vi "MainProgram.vi"() -> ()   [LabVIEW 2012]
uses:
  <vilib>/vision/Image Controls.llb/IMAQ Image.ctl
panel:
  out "error out 3":errorcluster
  out "error out 2":errorcluster
  out "error out":errorcluster
  in  "Tab Control":enum32{"MainProgram", ""}(tab)
  in  "Start Button":bool
  out "Judgment Failed":bool
  out "Image Out 2":T1(plugin-control)
  out "Red Found":i32
  out "R Score":sgl
  out "Red Status":bool
  in  "R Min Score":sgl=650.0
  in  "R Upper":dbl
  in  "R Lower":dbl
  in  "G Min score":sgl=800.0
  in  "G Upper":dbl
  in  "G Lower":dbl
  out "Green Status":bool
  out "G Score":sgl
  out "Green Found":i32
  out "Blue Status":bool
  out "Blue Found":i32
  out "B Score":sgl
  in  "B Min score":sgl=650.0
  in  "B Upper":dbl
  in  "B Lower":dbl
  out "Yellow Status":bool
  out "Yellow Found":i32
  out "Y Score":sgl
  in  "Y Min score":sgl=650.0
  in  "Y Upper":dbl
  in  "Y Lower":dbl
  out "Judgment Passed":bool
  in  "Stop (F)":bool
  out "Image Out 4":T1
  out "Image Out":T1(plugin-control)
  # "Check Fuse (Ver.1)"
  # "Test Result"
  # "Pass"
  # "Fail"
  # "Red Fuse"
  # "Green Fuse"
  # "Blue Fuse"
  # "Yellow Fuse"
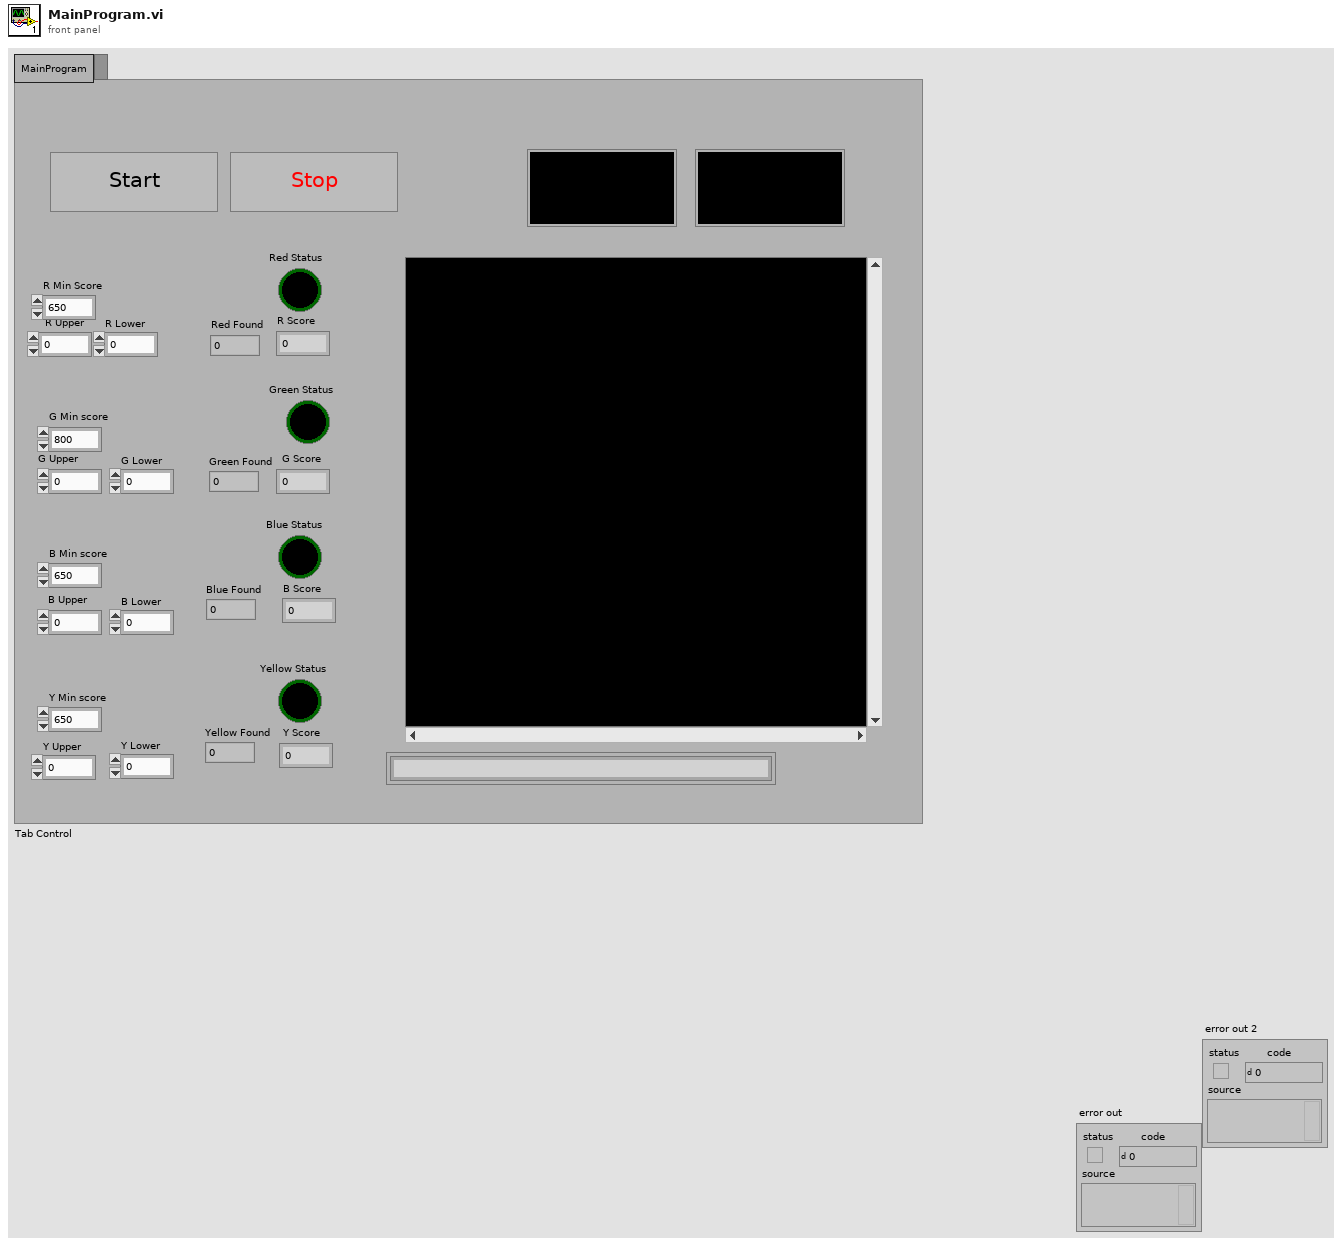
[diagram p1: front panel]
types:
  T1 = typedef "IMAQ Image.ctl" = refnum<image>
  T2 = cluster{"Desired Font (Application)":enum16{"User-specified Font", "Application Font", "System Font", "Dialog Font"}, "[User-specified Font]":cluster{"Font Name":string, "Size":i16, "Strikeout?":bool, "Italic?":bool, "Underline?":bool, "Outline?":bool, "Shadow?":bool, "Bold?":bool, "Rotation Angle":dbl}, "Horizontal Alignment":i16, "Vertical Alignment":i16}
  T3 = cluster{"Position":cluster{"x":sgl, "y":sgl}, "Angle":sgl, "Scale":sgl, "Score":sgl, "Bounding Box":cluster{"x":sgl, "y":sgl}[]}[]
  T4 = cluster{"Position":cluster{"x":sgl, "y":sgl}, "Angle":sgl, "Scale":sgl, "Score":sgl, "Bounding Box":cluster{"x":sgl, "y":sgl}[]}
  T5 = cluster{"Image Out":T1, "Image Out":T1, "Image Out":T1, "Image Out":T1, "Image Out":T1, "Image Out":T1, "Image Out":T1, "Image Out":T1}
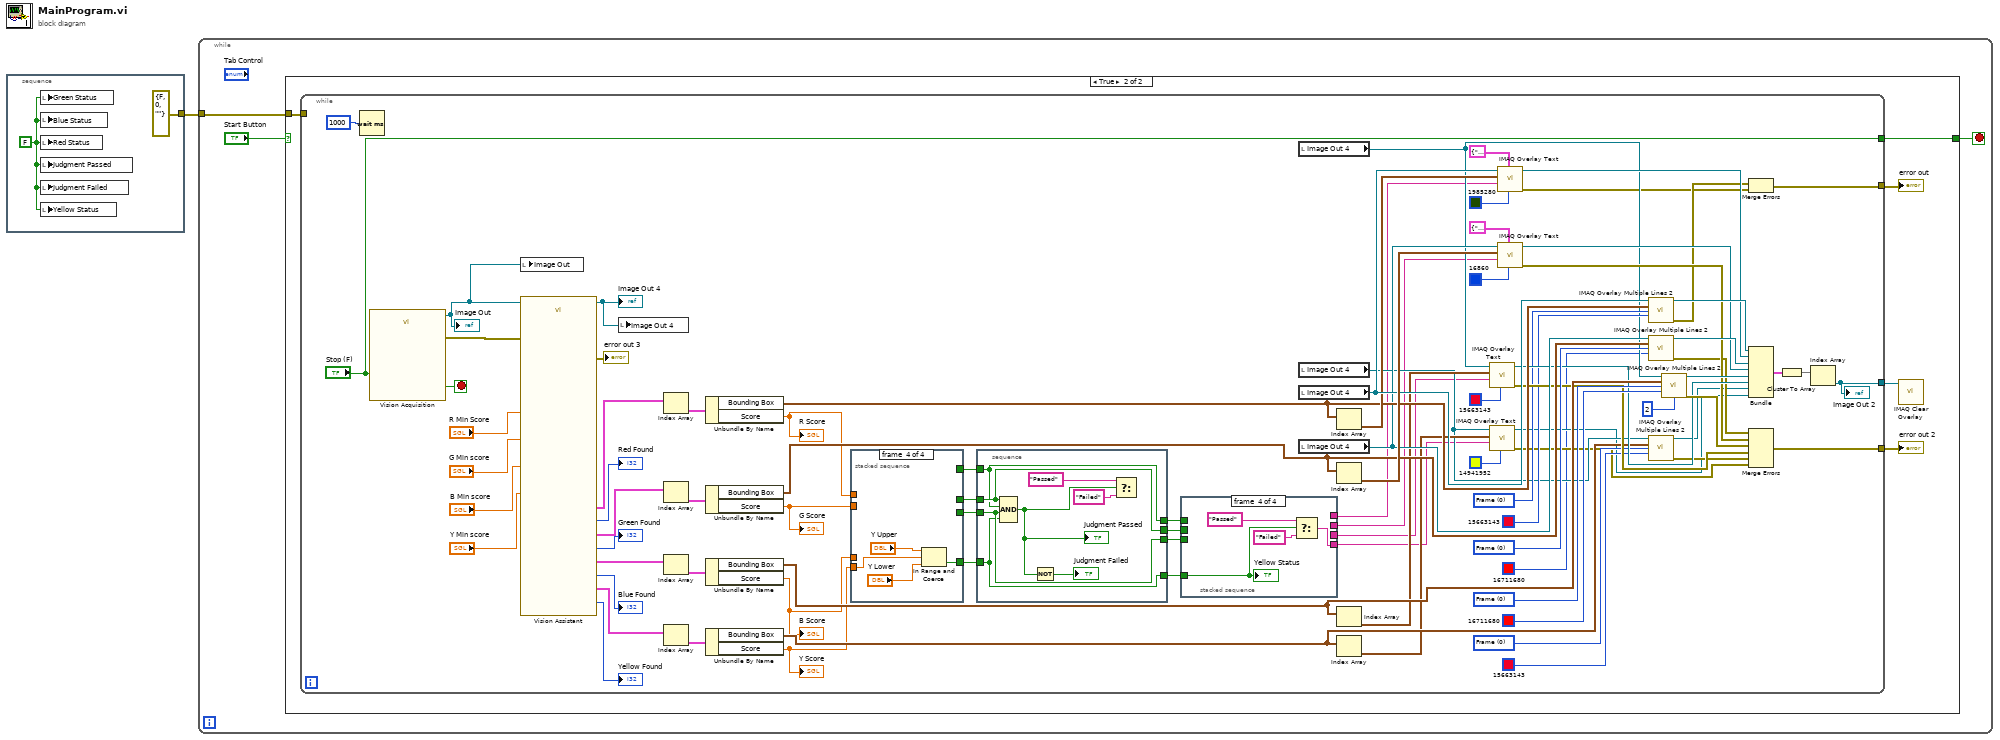
[diagram p0: block diagram]
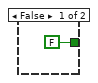
[diagram p2: hidden frame]
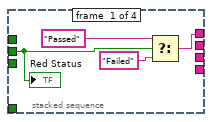
[diagram p3: hidden frame]
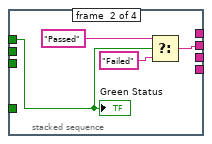
[diagram p4: hidden frame]
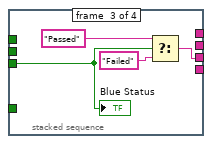
[diagram p5: hidden frame]
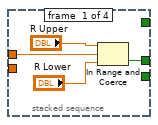
[diagram p6: hidden frame]
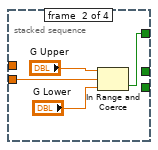
[diagram p7: hidden frame]
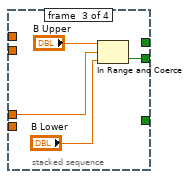
[diagram p8: hidden frame]
diagram:
  n1 = stacked-sequence {
    tunnel: [errorcluster {"status"=FALSE, "code"=0, "source"=""} ("error constant")] -> w1
    frame #0 {
      w3 = FALSE
      n2 = local write "Green Status"(w3) -> ()
      n3 = local write "Blue Status"(w3) -> ()
      n4 = local write "Red Status"(w3) -> ()
      n5 = local write "Judgment Passed"(w3) -> ()
      n6 = local write "Judgment Failed"(w3) -> ()
      n7 = local write "Yellow Status"(w3) -> ()
    }
  }
  n8 = while {
    tunnel: w1 -> [w4]
    stop <- w5 stop-if-true
    n9 = case shown="True" "Start Button" {
      tunnel: [FALSE ("Stop (F)") w11] -> w5
      tunnel: w4 -> [_ w8]
      frame False {
      }
      frame True {
        n10 = while {
          tunnel: [w97] -> w12
          tunnel: ["Stop (F)"] -> w11
          tunnel: [w17] -> w10
          tunnel: [w18] -> w9
          tunnel: w8 -> [_]
          stop <- w99 stop-if-true
          w48 = u32 0 items=["Frame", "Fill"] ("Drawing Mode (Frame)")
          w56 = u32 0 items=["Frame", "Fill"] ("Drawing Mode (Frame)")
          w68 = u32 0 items=["Frame", "Fill"] ("Drawing Mode (Frame)")
          w89 = u32 0 items=["Frame", "Fill"] ("Drawing Mode (Frame)")
          n11 = Wait (ms)(milliseconds to wait=u32 1000 ("millisecond multiple")) -> ()  [unwired: 1 out]
          n12 = call "Vision Acquisition"("Stop (F)"="Stop (F)") -> ("Image Out"=w96:T1, "Stopped"=w99:bool, "error out"=w14:errorcluster)  [unwired: 24 in]
          "Image Out" <- w96
          n13 = local write "Image Out"(w96) -> ()
          n14 = call "Vision Assistant"("Image In"=w96, "Minimum Match Score (Color Pattern Matching 3)"="B Min score", "Minimum Match Score (Color Pattern Matching 1)"="R Min Score", "error in"=w14, "Minimum Match Score (Color Pattern Matching 2)"="G Min score", "Minimum Match Score (Color Pattern Matching 4)"="Y Min score") -> ("Number of Matches (Color Pattern Matching 4)"=→"Yellow Found":i32, "Calibrated Matches (Color Pattern Matching 4)"=w52:T3, "Image Out"=w90:T1, "Calibrated Matches (Color Pattern Matching 1)"=w93:T3, "Number of Matches (Color Pattern Matching 1)"=→"Red Found":i32, "Calibrated Matches (Color Pattern Matching 2)"=w84:T3, "Number of Matches (Color Pattern Matching 2)"=→"Green Found":i32, "Calibrated Matches (Color Pattern Matching 3)"=w70:T3, "Number of Matches (Color Pattern Matching 3)"=→"Blue Found":i32, "error out"=→"error out 3":errorcluster)  [unwired: 12 in]
          "Image Out 4" <- w90
          n15 = local write "Image Out 4"(w90) -> ()
          n16 = Index Array(array=w93) -> (element=w95:T4)  [unwired: 1 in]
          n17 = Index Array(array=w84) -> (element=w73:T4)  [unwired: 1 in]
          n18 = Index Array(array=w70) -> (element=w69:T4)  [unwired: 1 in]
          n19 = Index Array(array=w52) -> (element=w51:T4)  [unwired: 1 in]
          n20 = Unbundle By Name(w95) -> ("Bounding Box"=w83:cluster{"x":sgl, "y":sgl}[], "Score"=w37:sgl)
          "R Score" <- w37
          n21 = Unbundle By Name(w73) -> ("Bounding Box"=w88:cluster{"x":sgl, "y":sgl}[], "Score"=w34:sgl)
          "G Score" <- w34
          n22 = Unbundle By Name(w69) -> ("Bounding Box"=w63:cluster{"x":sgl, "y":sgl}[], "Score"=w32:sgl)
          "B Score" <- w32
          n23 = Unbundle By Name(w51) -> ("Bounding Box"=w44:cluster{"x":sgl, "y":sgl}[], "Score"=w30:sgl)
          "Y Score" <- w30
          n24 = stacked-sequence {
            tunnel: w37 -> [w125 _ _ _]
            tunnel: [w124 _ _ _] -> w36
            tunnel: [_ w129 _ _] -> w35
            tunnel: w34 -> [_ w128 _ _]
            tunnel: [_ _ w133 _] -> w33
            tunnel: w32 -> [_ _ w132 _]
            tunnel: [_ _ _ w137] -> w31
            tunnel: w30 -> [_ _ _ w136]
            frame #0 {
              n25 = In Range and Coerce(upper limit="R Upper", x=w125, lower limit="R Lower") -> (In Range?=w124:bool)  [unwired: 1 out]
            }
            frame #1 {
              n26 = In Range and Coerce(upper limit="G Upper", x=w128, lower limit="G Lower") -> (In Range?=w129:bool)  [unwired: 1 out]
            }
            frame #2 {
              n27 = In Range and Coerce(upper limit="B Upper", x=w132, lower limit="B Lower") -> (In Range?=w133:bool)  [unwired: 1 out]
            }
            frame #3 {
              n28 = In Range and Coerce(upper limit="Y Upper", x=w136, lower limit="Y Lower") -> (In Range?=w137:bool)  [unwired: 1 out]
            }
          }
          n29 = stacked-sequence {
            tunnel: w36 -> [w121]
            tunnel: w35 -> [w120]
            tunnel: w33 -> [w119]
            tunnel: w31 -> [w118]
            tunnel: [w121] -> w29
            tunnel: [w120] -> w27
            tunnel: [w119] -> w25
            tunnel: [w118] -> w23
            frame #0 {
              n30 = Compound Arithmetic op=AND(w121, w120, w119, w118) -> (w117:bool)
              "Judgment Passed" <- w117
              n31 = Not(x=w117) -> (.not. x?=→"Judgment Failed":bool)
              n32 = Select(t="Passed", s=w117, f="Failed") -> ()  [unwired: 1 out]
            }
          }
          n33 = stacked-sequence {
            tunnel: w29 -> [w100 _ _ _]
            tunnel: [w102 _ _ _] -> w28
            tunnel: w27 -> [_ w105 _ _]
            tunnel: [_ w104 _ _] -> w26
            tunnel: w25 -> [_ _ w109 _]
            tunnel: [_ _ w108 _] -> w24
            tunnel: w23 -> [_ _ _ w112]
            tunnel: [_ _ _ w113] -> w22
            frame #0 {
              n34 = Select(t="Passed", s=w100, f="Failed" ("t")) -> (s? t:f=w102:string)
              "Red Status" <- w100
            }
            frame #1 {
              n35 = Select(t="Passed", s=w105, f="Failed" ("t")) -> (s? t:f=w104:string)
              "Green Status" <- w105
            }
            frame #2 {
              n36 = Select(t="Passed", s=w109, f="Failed" ("t")) -> (s? t:f=w108:string)
              "Blue Status" <- w109
            }
            frame #3 {
              n37 = Select(t="Passed", s=w112, f="Failed" ("t")) -> (s? t:f=w113:string)
              "Yellow Status" <- w112
            }
          }
          n38 = local read "Image Out 4"() -> (w49:T1)
          n39 = local read "Image Out 4"() -> (w42:T1)
          n40 = local read "Image Out 4"() -> (w87:T1)
          n41 = local read "Image Out 4"() -> (w72:T1)
          n42 = Index Array(array=w83) -> (element=w86:cluster{"x":sgl, "y":sgl})  [unwired: 1 in]
          n43 = Index Array(array=w88) -> (element=w92:cluster{"x":sgl, "y":sgl})  [unwired: 1 in]
          n44 = Index Array(array=w63) -> (element=w62:cluster{"x":sgl, "y":sgl})  [unwired: 1 in]
          n45 = Index Array(array=w44) -> (element=w43:cluster{"x":sgl, "y":sgl})  [unwired: 1 in]
          n46 = call "IMAQ Overlay Text"("Text Color (black)"=u32 15663143, "String"=w24, "Origin"=w62, "Image"=w49) -> ("error out"=w59:errorcluster, "Image Out"=w60:T1)  [unwired: 6 in]
          n47 = call "IMAQ Overlay Text"("Text Color (black)"=u32 14941952, "String"=w22, "Origin"=w43, "Image"=w42) -> ("error out"=w40:errorcluster, "Image Out"=w39:T1)  [unwired: 6 in]
          n48 = call "IMAQ Overlay Text"("Text Color (black)"=u32 1985280, "Font, Size & Style"=T2 {"Desired Font (Application)"=enum."Application Font", "[User-specified Font]"={"Font Name"="", "Size"=30, "Strikeout?"=FALSE, "Italic?"=FALSE, "Underline?"=FALSE, "Outline?"=FALSE, "Shadow?"=FALSE, "Bold?"=FALSE, "Rotation Angle"=0.0}, "Horizontal Alignment"=0, "Vertical Alignment"=0}, "String"=w28, "Origin"=w86, "Image"=w87) -> ("error out"=w15:errorcluster, "Image Out"=w81:T1)  [unwired: 5 in]
          n49 = call "IMAQ Overlay Text"("Text Color (black)"=u32 16860, "Font, Size & Style"=T2 {"Desired Font (Application)"=enum."Application Font", "[User-specified Font]"={"Font Name"="", "Size"=30, "Strikeout?"=FALSE, "Italic?"=FALSE, "Underline?"=FALSE, "Outline?"=FALSE, "Shadow?"=FALSE, "Bold?"=FALSE, "Rotation Angle"=0.0}, "Horizontal Alignment"=0, "Vertical Alignment"=0}, "String"=w26, "Origin"=w92, "Image"=w72) -> ("error out"=w54:errorcluster, "Image Out"=w79:T1)  [unwired: 5 in]
          n50 = call "IMAQ Overlay Multiple Lines 2"("Image"=w87, "Line End Points"=w83, "Drawing Mode (Frame)"=w56, "Color"=u32 15663143) -> ("Image Out"=w82:T1, "error out"=w16:errorcluster)  [unwired: 10 in]
          n51 = call "IMAQ Overlay Multiple Lines 2"("Image"=w72, "Line End Points"=w88, "Drawing Mode (Frame)"=w89, "Color"=u32 16711680) -> ("Image Out"=w80:T1, "error out"=w53:errorcluster)  [unwired: 10 in]
          n52 = call "IMAQ Overlay Multiple Lines 2"("Image"=w42, "Line End Points"=w44, "Drawing Mode (Frame)"=w48, "Color"=u32 15663143) -> ("Image Out"=w46:T1, "error out"=w45:errorcluster)  [unwired: 10 in]
          n53 = call "IMAQ Overlay Multiple Lines 2"("Image"=w49, "Line End Points"=w63, "Drawing Mode (Frame)"=w68, "Color"=u32 16711680, "Width"=u32 2) -> ("Image Out"=w65:T1, "error out"=w64:errorcluster)  [unwired: 9 in]
          n54 = Merge Errors(w16, w15) -> (w17:errorcluster)
          n55 = Bundle("Image Out"=w82, "Image Out"=w81, "Image Out"=w80, "Image Out"=w79, "Image Out"=w65, "Image Out"=w60, "Image Out"=w46, "Image Out"=w39) -> (w78:T5)  [unwired: 1 in]
          n56 = Merge Errors(w53, w54, w64, w59, w45, w40) -> (w18:errorcluster)
          n57 = Cluster To Array(cluster=w78) -> (array=w77:T1[])
          n58 = Index Array(array=w77) -> (element=w97:T1)  [unwired: 1 in]
          "Image Out 2" <- w97
        }
        "error out" <- w10
        "error out 2" <- w9
        n59 = call "IMAQ Clear Overlay"("Image"=w12) -> ()  [unwired: 9 in, 2 out]
      }
    }
  }
